vi "Data.Create.vi"(6 "Type":enum16{"Read", "Write", "ReadWrite"}(ring), 7 "Name":string, 8 "error in (no error)":errorcluster, 9 "Channel Refs":T1[](array[typedef]) format="%.0x", 10 "Custom Device Ref":T1 format="%.0x", 11 "Data Access API in":refnum<class "Data Access API.lvclass">) -> (0 "error out":errorcluster, 2 "Custom Device Ref out":T1 format="%.0x", 3 "Data Access API out":refnum<class "Data Access API.lvclass">)   [LabVIEW 2015, in "Data Access API.lvlib" / "Data Access API.lvclass"]
uses:
  Data Access API.lvclass
  <vilib>/NI Veristand/Custom Device API/Custom Device Item Ref.ctl
  Data/Read/Read.lvclass
  Data Access API.lvclass/Data Access API.ctl
  Data/Read/Read.lvclass/Read.ctl
  Data/Write/Write.lvclass
  Data/Write/Write.lvclass/Write.ctl
  Data/ReadWrite/ReadWrite.lvclass
  Data/ReadWrite/ReadWrite.lvclass/ReadWrite.ctl
  <vilib>/NI Veristand/Custom Device API/NI VeriStand - Get Channel Data Reference.vi
  <vilib>/NI Veristand/Custom Device API/NI VeriStand - Get Custom Device Channel Data.vi
  <vilib>/NI Veristand/Custom Device API/NI VeriStand - Get Channel Block Data References.vi
  <vilib>/NI Veristand/Custom Device API/Custom Device API.lvlib
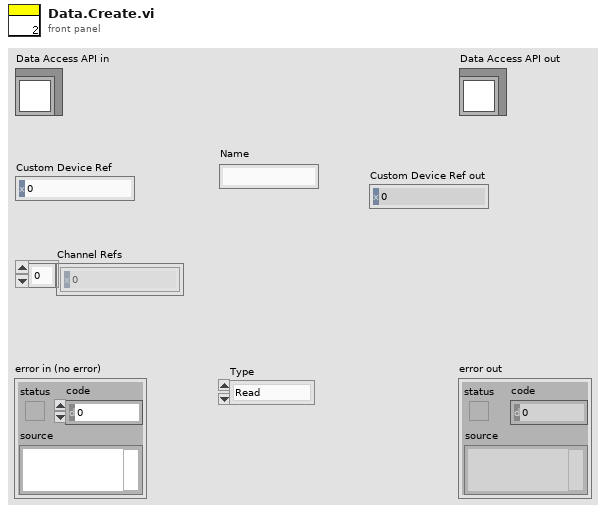
[diagram p1: front panel]
types:
  T1 = typedef "Custom Device API.lvlib/Custom Device Item Ref.ctl" = u64
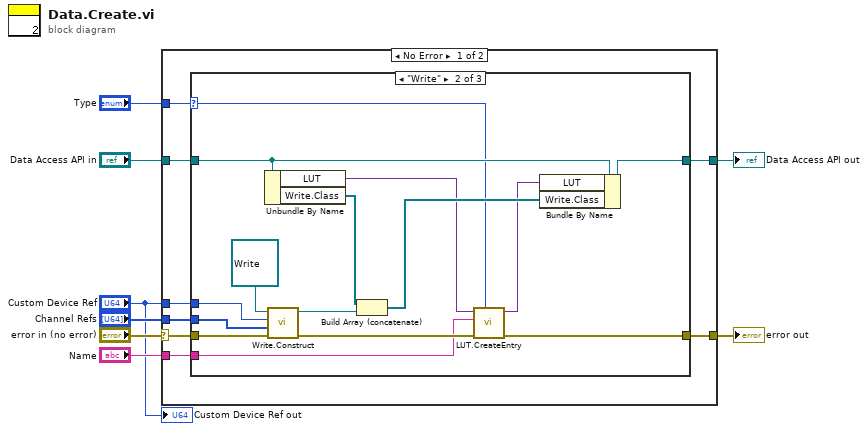
[diagram p0: block diagram]
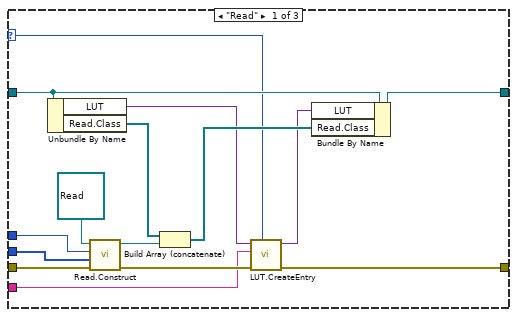
[diagram p2: hidden frame]
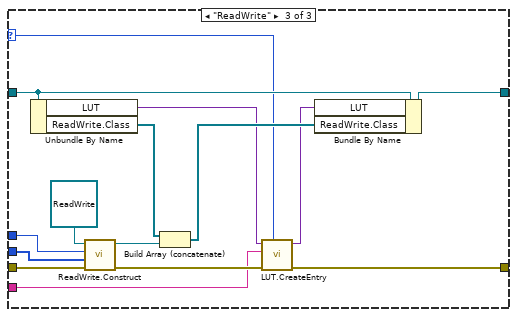
[diagram p3: hidden frame]
diagram:
  n1 = case shown="No Error" "error in (no error)" {
    selector: "error in (no error)" -> [w13 w63]
    tunnel: [w12 w63] -> w7
    tunnel: [w14 w62] -> w5
    tunnel: "Data Access API in" -> [w15 w62]
    tunnel: "Type" -> [w16 _]
    tunnel: "Channel Refs" -> [w11 _]
    tunnel: "Custom Device Ref" -> [w10 _]
    tunnel: "Name" -> [w9 _]
    frame No Error {
      n2 = case shown="\"Write\"" w16 {
        selector: w16 -> [w18 w35 w49]
        tunnel: w15 -> [w29 w43 w60]
        tunnel: [w28 w42 w59] -> w14
        tunnel: w13 -> [w26 w41 w57]
        tunnel: [w21 w36 w50] -> w12
        tunnel: w11 -> [w24 w39 w56]
        tunnel: w10 -> [w25 w40 w55]
        tunnel: w9 -> [w17 w34 w47]
        frame "Read" {
          n3 = Unbundle By Name(w29) -> ("LUT"=w20:variant, "Read.Class"=w31:refnum<class "Read.lvclass">[])
          n4 = call "Read.Construct.vi"("error in (no error)"=w26, "Refs"=w24, "Parent"=w25, "Read in"=refnum<class "Read.lvclass"> refnum ("Read.lvclass")) -> ("error out"=w22:errorcluster, "Read out"=w23:refnum<class "Read.lvclass">)  [unwired: 6 in]
          n5 = Build Array (concatenate)(w31, w23) -> (w30:refnum<class "Read.lvclass">[])
          n6 = call "LUT.CreateEntry.vi"("Type"=w18, "error in (no error)"=w22, "Name"=w17, "LUT"=w20) -> ("error out"=w21:errorcluster, "LUT"=w19:variant)  [unwired: 6 in]
          n7 = Bundle By Name(cluster=w29, "LUT"=w19, "Read.Class"=w30) -> (w28:refnum<class "Data Access API.lvclass">)
        }
        frame "Write" {
          n8 = Unbundle By Name(w43) -> ("LUT"=w33:variant, "Write.Class"=w45:refnum<class "Write.lvclass">[])
          n9 = call "Write.Construct.vi"("error in (no error)"=w41, "Refs"=w39, "Parent"=w40, "Write in"=refnum<class "Write.lvclass"> refnum ("Write.lvclass")) -> ("error out"=w37:errorcluster, "Write out"=w38:refnum<class "Write.lvclass">)  [unwired: 6 in]
          n10 = Build Array (concatenate)(w45, w38) -> (w44:refnum<class "Write.lvclass">[])
          n11 = call "LUT.CreateEntry.vi"("Type"=w35, "error in (no error)"=w37, "Name"=w34, "LUT"=w33) -> ("error out"=w36:errorcluster, "LUT"=w32:variant)  [unwired: 6 in]
          n12 = Bundle By Name(cluster=w43, "LUT"=w32, "Write.Class"=w44) -> (w42:refnum<class "Data Access API.lvclass">)
        }
        frame "ReadWrite" {
          n13 = Unbundle By Name(w60) -> ("LUT"=w48:variant, "ReadWrite.Class"=w61:refnum<class "ReadWrite.lvclass">[])
          n14 = call "ReadWrite.Construct.vi"("error in (no error)"=w57, "Refs"=w56, "Parent"=w55, "ReadWrite in"=refnum<class "ReadWrite.lvclass"> refnum ("ReadWrite.lvclass")) -> ("error out"=w51:errorcluster, "ReadWrite out"=w54:refnum<class "ReadWrite.lvclass">)  [unwired: 6 in]
          n15 = Build Array (concatenate)(w61, w54) -> (w53:refnum<class "ReadWrite.lvclass">[])
          n16 = call "LUT.CreateEntry.vi"("Type"=w49, "error in (no error)"=w51, "Name"=w47, "LUT"=w48) -> ("error out"=w50:errorcluster, "LUT"=w52:variant)  [unwired: 6 in]
          n17 = Bundle By Name(cluster=w60, "LUT"=w52, "ReadWrite.Class"=w53) -> (w59:refnum<class "Data Access API.lvclass">)
        }
      }
    }
    frame Error {
    }
  }
  "error out" <- w7
  "Data Access API out" <- w5
  "Custom Device Ref out" <- "Custom Device Ref"
